vi "RSMStamps.vi"(0 "Sequence Context In":refnum<k7>, 7 "error IN":errorcluster) -> (20 "Sequence Context Out":refnum<k7>, 21 "FilePath":string, 22 "TimeStamp":string, 23 "DateStamp":string, 24 "SerialNumber":string, 25 "ModelNumber":string, 27 "error Out":errorcluster)   [LabVIEW 2014]
uses:
  <vilib>/addons/TestStand/_TSUtility.llb/TestStand - Get Property Value (String).vi
  <vilib>/addons/TestStand/_TSUtility.llb/TestStand - Get Property Value (Number).vi
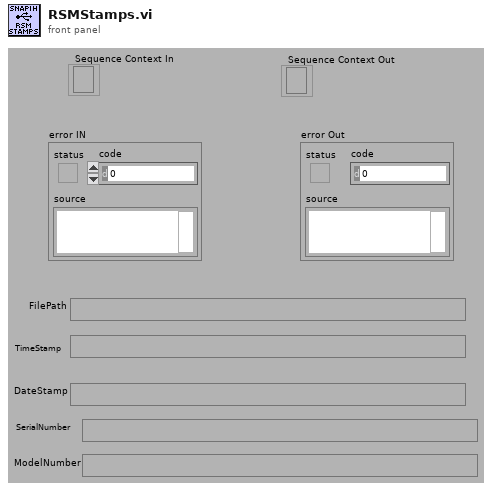
[diagram p1: front panel]
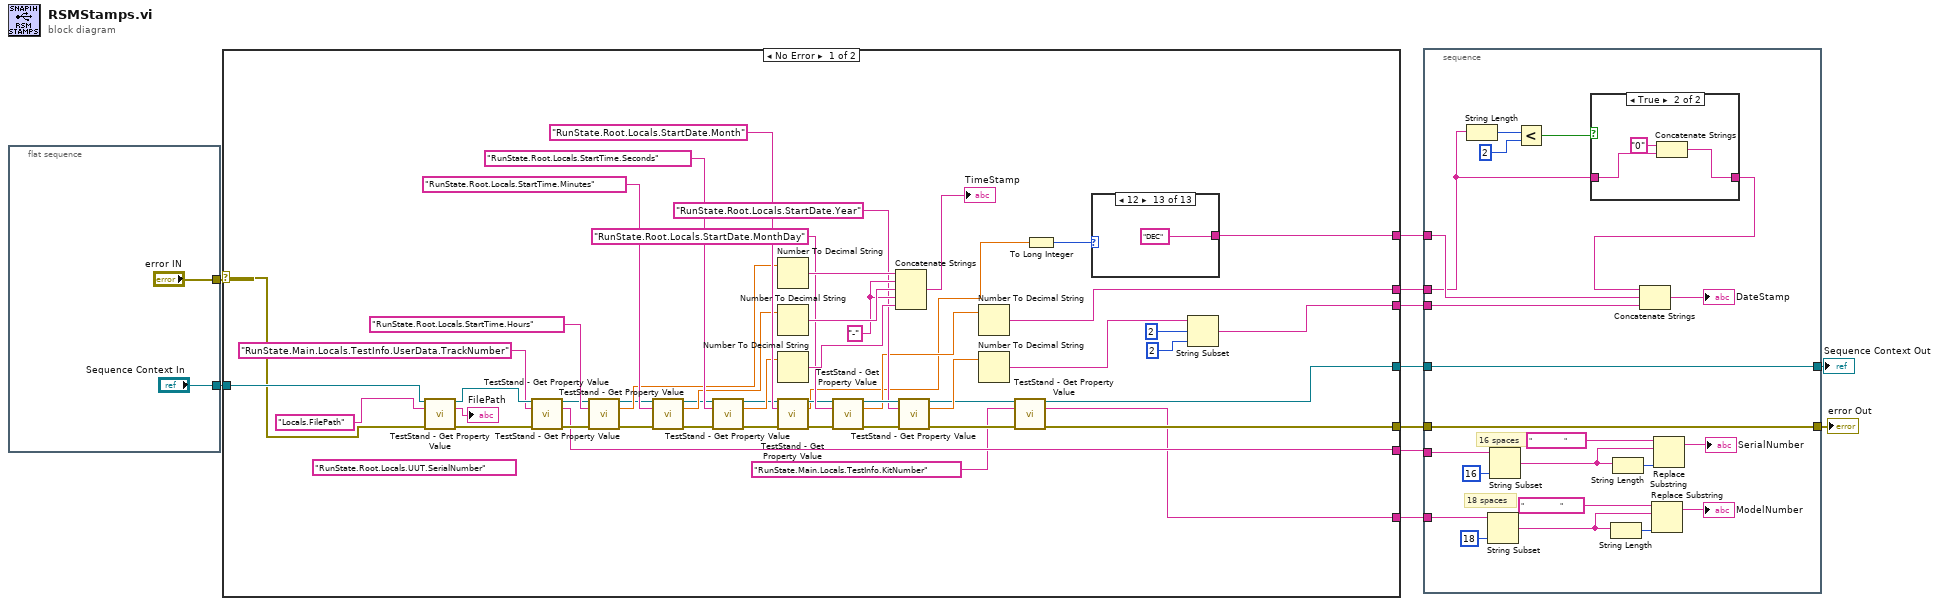
[diagram p0: block diagram]
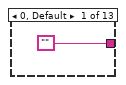
[diagram p3: hidden frame]
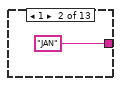
[diagram p4: hidden frame]
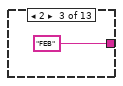
[diagram p5: hidden frame]
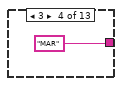
[diagram p6: hidden frame]
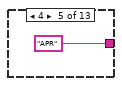
[diagram p7: hidden frame]
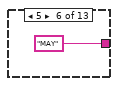
[diagram p8: hidden frame]
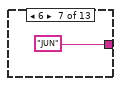
[diagram p9: hidden frame]
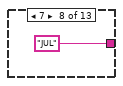
[diagram p10: hidden frame]
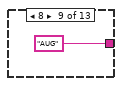
[diagram p11: hidden frame]
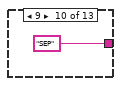
[diagram p12: hidden frame]
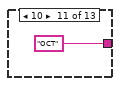
[diagram p13: hidden frame]
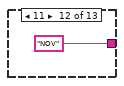
[diagram p14: hidden frame]
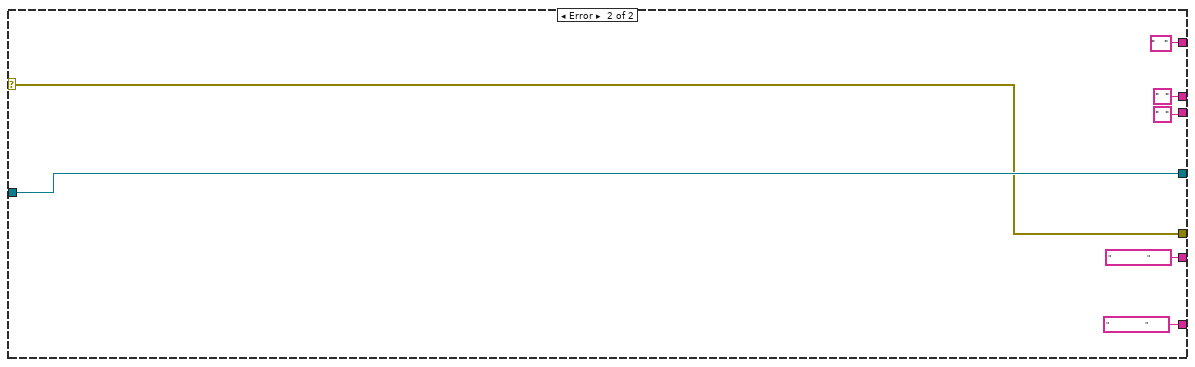
[diagram p15: hidden frame]
diagram:
  n1 = flat-sequence {
    tunnel: ["Sequence Context In"] -> w11
    tunnel: ["error IN"] -> w10
    frame #0 {
    }
  }
  n2 = case shown="No Error" w10 {
    selector: w10 -> [w30 w82]
    tunnel: [w16 w82] -> w7
    tunnel: [w15 w83] -> w9
    tunnel: w11 -> [w56 w83]
    tunnel: [w25 "   "] -> w5
    tunnel: [w26 "  "] -> w4
    tunnel: [w20 "  "] -> w3
    tunnel: [w24 "                  " ("Value")] -> w2
    tunnel: [w14 "                  "] -> w1
    frame No Error {
      (unwired) "RunState.Root.Locals.UUT.SerialNumber" ("Lookup String")
      w41 = "-" ("string")
      n3 = call-poly <vilib>:"TestStand - Get Property Value.vi"("Sequence Context In"=w56, "Lookup String"="Locals.FilePath", "error in (no error)"=w30) -> ("Sequence Context Out"=w61:refnum<k7>, "Value"=→"FilePath":string, "error out"=w62:errorcluster)  [unwired: 10 in]
      n4 = call-poly <vilib>:"TestStand - Get Property Value.vi"("Sequence Context In"=w61, "Lookup String"="RunState.Main.Locals.TestInfo.UserData.TrackNumber", "error in (no error)"=w62) -> ("Sequence Context Out"=w53:refnum<k7>, "Value"=w24:string, "error out"=w63:errorcluster)  [unwired: 10 in]
      n5 = call-poly <vilib>:"TestStand - Get Property Value.vi"("Sequence Context In"=w53, "Lookup String"="RunState.Root.Locals.StartTime.Hours", "error in (no error)"=w63) -> ("Sequence Context Out"=w49:refnum<k7>, "Value"=w52:dbl, "error out"=w46:errorcluster)  [unwired: 10 in]
      n6 = call-poly <vilib>:"TestStand - Get Property Value.vi"("Sequence Context In"=w49, "Lookup String"="RunState.Root.Locals.StartTime.Minutes", "error in (no error)"=w46) -> ("Sequence Context Out"=w48:refnum<k7>, "Value"=w51:dbl, "error out"=w45:errorcluster)  [unwired: 10 in]
      n7 = call-poly <vilib>:"TestStand - Get Property Value.vi"("Sequence Context In"=w48, "Lookup String"="RunState.Root.Locals.StartTime.Seconds", "error in (no error)"=w45) -> ("Sequence Context Out"=w47:refnum<k7>, "Value"=w50:dbl, "error out"=w44:errorcluster)  [unwired: 10 in]
      n8 = Number To Decimal String(number=w52) -> (decimal integer string=w43:string)  [unwired: 1 in]
      n9 = Number To Decimal String(number=w51) -> (decimal integer string=w42:string)  [unwired: 1 in]
      n10 = Number To Decimal String(number=w50) -> (decimal integer string=w40:string)  [unwired: 1 in]
      n11 = call-poly <vilib>:"TestStand - Get Property Value.vi"("Sequence Context In"=w47, "Lookup String"="RunState.Root.Locals.StartDate.Month", "error in (no error)"=w44) -> ("Sequence Context Out"=w37:refnum<k7>, "Value"=w28:dbl, "error out"=w36:errorcluster)  [unwired: 10 in]
      n12 = call-poly <vilib>:"TestStand - Get Property Value.vi"("Sequence Context In"=w37, "Lookup String"="RunState.Root.Locals.StartDate.MonthDay", "error in (no error)"=w36) -> ("Sequence Context Out"=w34:refnum<k7>, "Value"=w32:dbl, "error out"=w35:errorcluster)  [unwired: 10 in]
      n13 = Concatenate Strings(w43, w41, w42, w41, w40) -> (→"TimeStamp":string)
      n14 = call-poly <vilib>:"TestStand - Get Property Value.vi"("Sequence Context In"=w34, "Lookup String"="RunState.Root.Locals.StartDate.Year", "error in (no error)"=w35) -> ("Sequence Context Out"=w18:refnum<k7>, "Value"=w31:dbl, "error out"=w19:errorcluster)  [unwired: 10 in]
      n15 = Number To Decimal String(number=w32) -> (decimal integer string=w26:string)  [unwired: 1 in]
      n16 = Number To Decimal String(number=w31) -> (decimal integer string=w23:string)  [unwired: 1 in]
      n17 = call-poly <vilib>:"TestStand - Get Property Value.vi"("Sequence Context In"=w18, "Lookup String"="RunState.Main.Locals.TestInfo.KitNumber", "error in (no error)"=w19) -> ("Sequence Context Out"=w15:refnum<k7>, "Value"=w14:string, "error out"=w16:errorcluster)  [unwired: 10 in]
      n18 = To Long Integer(number=w28) -> (32bit integer=w27:i32)
      n19 = case shown="12" w27 {
        tunnel: ["" "JAN" ("Month") "FEB" ("Month") "MAR" ("Month") "APR" ("Month") "MAY" ("Month") "JUN" ("Month") "JUL" ("Month") "AUG" ("Month") "SEP" ("Month") "OCT" ("Month") "NOV" ("Month") "DEC" ("Month")] -> w25
        frame 0, Default {
        }
        frame 1 {
        }
        frame 2 {
        }
        frame 3 {
        }
        frame 4 {
        }
        frame 5 {
        }
        frame 6 {
        }
        frame 7 {
        }
        frame 8 {
        }
        frame 9 {
        }
        frame 10 {
        }
        frame 11 {
        }
        frame 12 {
        }
      }
      n20 = String Subset(string=w23, offset (0)=2, length (rest)=2 ("length (rest)")) -> (substring=w20:string)
    }
    frame Error {
    }
  }
  n21 = stacked-sequence {
    tunnel: w9 -> [w105]
    tunnel: [w105] -> w8
    tunnel: w7 -> [w104]
    tunnel: [w104] -> w6
    tunnel: w5 -> [w86]
    tunnel: w4 -> [w85]
    tunnel: w3 -> [w102]
    tunnel: w2 -> [w98]
    tunnel: w1 -> [w90]
    frame #0 {
      # "18 spaces"
      # "16 spaces"
      n22 = String Length(string=w85) -> (length=w89:i32)
      n23 = String Subset(string=w90, length (rest)=18 ("length (rest)")) -> (substring=w92:string)  [unwired: 1 in]
      n24 = String Subset(string=w98, length (rest)=16 ("length (rest)")) -> (substring=w97:string)  [unwired: 1 in]
      n25 = Less?(x=w89, y=2) -> (x < y?=w87:bool)
      n26 = case shown="True" w87 {
        tunnel: w85 -> [w106 w108]
        tunnel: [w106 w107] -> w84
        frame False {
        }
        frame True {
          n27 = Concatenate Strings("0" ("string"), w108) -> (w107:string)
        }
      }
      n28 = String Length(string=w92) -> (length=w94:i32)
      n29 = String Length(string=w97) -> (length=w100:i32)
      n30 = Concatenate Strings(w84, w86, w102) -> (→"DateStamp":string)
      n31 = Replace Substring(2:w94, 4:w92, 5:"                  " ("string")) -> (1:→"ModelNumber":string)  [unwired: 1 in, 1 out]
      n32 = Replace Substring(2:w100, 4:w97, 5:"                " ("string")) -> (1:→"SerialNumber":string)  [unwired: 1 in, 1 out]
    }
  }
  "error Out" <- w6
  "Sequence Context Out" <- w8
